vi "CSP_CalculatePCA.vi"(11 "CSP.lvclass in":refnum<class "CSP.lvclass">) -> (3 "CSP.lvclass out":refnum<class "CSP.lvclass">)   [LabVIEW 2016, in "Spatial Pattern Filter.lvlib" / "CSP.lvclass"]
uses:
  CSP.lvclass
  CSP.lvclass/CSP.ctl
  <vilib>/Analysis/7linalg.llb/Real Eigenvalues and Vectors.vi
  <vilib>/Analysis/NI_AALPro.lvlib
  Spatial Pattern Filter.lvlib
panel:
  # "This VI is a part of BCI Design library, http://www.ru-bci.org \nCopyright © 2020, Sotnikov Peter, All rights reserved. License: GNU GPLv3"
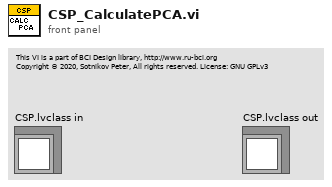
[diagram p1: front panel]
types:
  T1 = typedef "NI_Matrix.lvlib/RealMatrix.ctl" = dbl[][]
  T2 = cluster{"PCAMatrix":T1, "CovarianceMatrix":T1, "MeanValue":dbl[][]}[]
  T3 = typedef "NI_Matrix.lvlib/ComplexMatrix.ctl" = cdb[][]
  T4 = cluster{"PCAMatrix":T1, "CovarianceMatrix":T1, "MeanValue":dbl[][]}
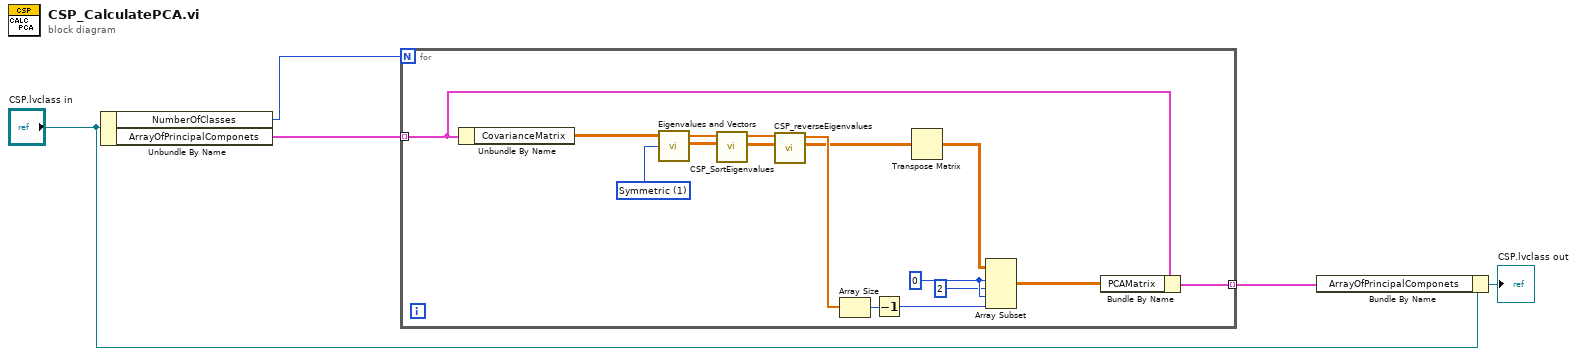
[diagram p0: block diagram]
diagram:
  n1 = Unbundle By Name("CSP.lvclass in") -> ("NumberOfClasses"=w5:i32, "ArrayOfPrincipalComponets"=w4:T2)
  n2 = for {
    N: w5 -> [_]
    tunnel: w4 -> [w10] mode=indexing
    tunnel: [w8] -> w2 mode=indexing
    w17 = 0 ("row 1")
    w20 = 1 items=["General", "Symmetric"] ("matrix type")
    n3 = Unbundle By Name(w10) -> ("CovarianceMatrix"=w21:T1)
    n4 = call-poly <vilib>:"Eigenvalues and Vectors.vi"("matrix type"=w20, "Input Matrix"=w21) -> ("Eigenvectors"=w18:T3, "Eigenvalues"=w19:cdb[])  [unwired: 1 in, 1 out]
    n5 = call "CSP_SortEigenvalues.vi"("Eigenvectors"=w18, "Eigenvalues"=w19) -> ("Eigenvectors Sorted"=w12:T3, "Eigenvalues Sorted"=w13:dbl[])  [unwired: 8 in]
    n6 = call "CSP_reverseEigenvalues.vi"("Eigenvectors in"=w12, "Eigenvalues in"=w13) -> ("Reversed Eigenvectors"=w7:T3, "Reversed Eigenvalues"=w11:cdb[])  [unwired: 6 in]
    n7 = Array Size(array=w11) -> (size(s)=w14:i32)
    n8 = Decrement(x=w14) -> (x-1=w15:i32)
    n9 = Transpose Matrix(1:w7) -> (0:w6:T3)
    n10 = Array Subset(array=w6, index (row)=w17, length (row)=2 ("row N"), index (col)=w17, length (col)=w15) -> (w9:T3)
    n11 = Bundle By Name(cluster=w10, "PCAMatrix"=w9) -> (w8:T4)
  }
  n12 = Bundle By Name(cluster="CSP.lvclass in", "ArrayOfPrincipalComponets"=w2) -> (→"CSP.lvclass out":refnum<class "CSP.lvclass">)
